vi "Adquisicio_projecte_InsEl (2).vi"() -> ()   [LabVIEW 2014]
uses:
  <vilib>/DAQmx/configure/timing.llb/DAQmx Timing (Sample Clock).vi
  <vilib>/DAQmx/read.llb/DAQmx Read (Analog 1D Wfm NChan NSamp).vi
panel:
  in  "V2":dbl
  in  "V1":dbl
  in  "T2":dbl
  in  "T1":dbl
  in  "Numero de Media":dbl
  in  "Durada adquisició":dbl
  in  "Temps entre adquisicions":dbl
  out "?":bool
  out "?":bool
  out "?":bool
  out "?":bool
  in  "CH 4":bool
  in  "CH 3":bool
  in  "CH 2":bool
  in  "CH 1":bool
  in  "?":bool
  in  "?":bool
  out "Registro Temperatura CH 4":dbl[](graph)
  out "Registro Temperatura CH 3":dbl[](graph)
  out "Registro Temperatura CH 2":dbl[](graph)
  out "Registro Temperatura CH 1":dbl[](graph)
  in  "Tab Control":enum32{"CH 1", "CH 2", "CH 3", "CH 4"}(tab)
  out "T min CH 1":dbl
  out "T max CH 1":dbl
  in  "T max CH 1":dbl
  in  "T min CH 1":dbl
  out "IND CH 1":u32(colorbox)
  out "H CH 1":dbl[](array[numeric])
  out "desviació 1":dbl
  in  "T max CH 2":dbl
  in  "T min CH 2":dbl
  out "IND CH 2":u32(colorbox)
  out "H CH 2":dbl[](array[numeric])
  out "T max CH 2":dbl
  out "T min CH 2":dbl
  in  "T max CH 3":dbl
  in  "T min CH 3":dbl
  out "IND CH 3":u32(colorbox)
  out "H CH 3":dbl[](array[numeric])
  out "T max CH 3":dbl
  out "T min CH 3":dbl
  out "Desviació 3":dbl
  in  "T max CH 4":dbl
  in  "T min CH 4":dbl
  out "IND CH 4":u32(colorbox)
  out "H CH 4":dbl[](array[numeric])
  out "T max CH 4":dbl
  out "T min CH 4":dbl
  out "Desviació 4":dbl
  in  "PARAR PROGRAMA":bool
  out "MEDIA CH 4":dbl
  out "MEDIA CH 3":dbl
  out "MEDIA CH 2":dbl
  out "MEDIA CH 1":dbl
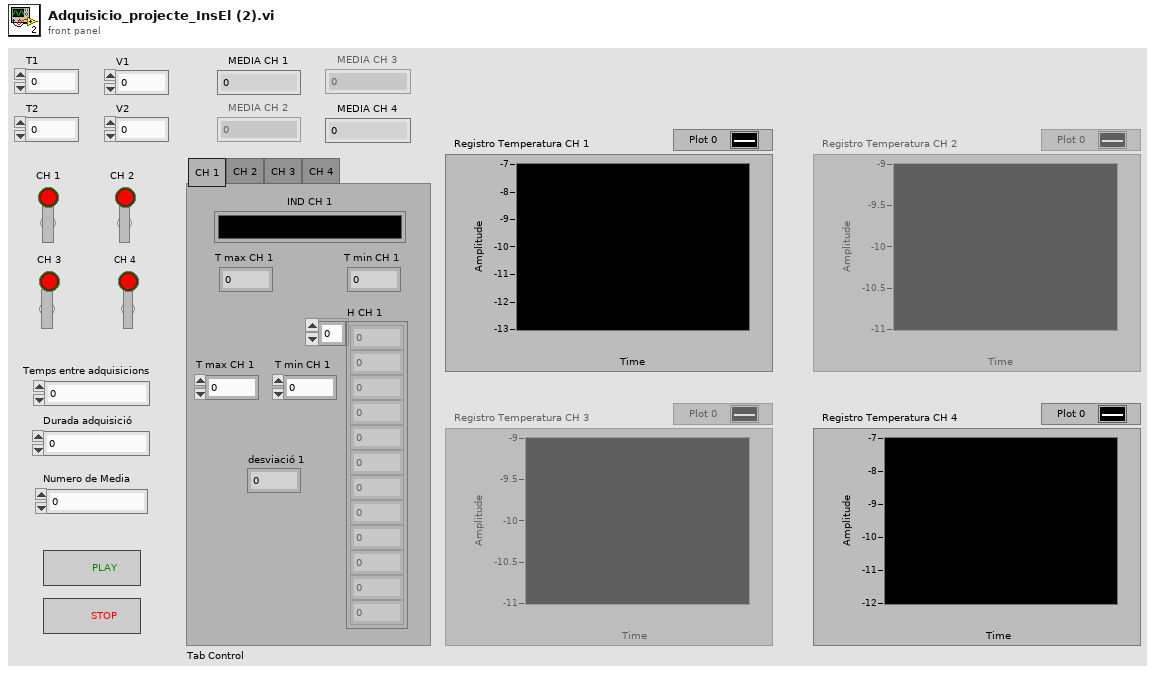
[diagram p1: front panel]
types:
  T1 = enum16{"open", "replace", "create", "open or create", "replace or create", "replace or create with confirmation"}
  T2 = enum8{"Enabled", "Disabled", "Disabled and Grayed Out"}
  T3 = cluster{"CH 1":bool, "CH 2":bool, "CH 3":bool, "CH 4":bool}
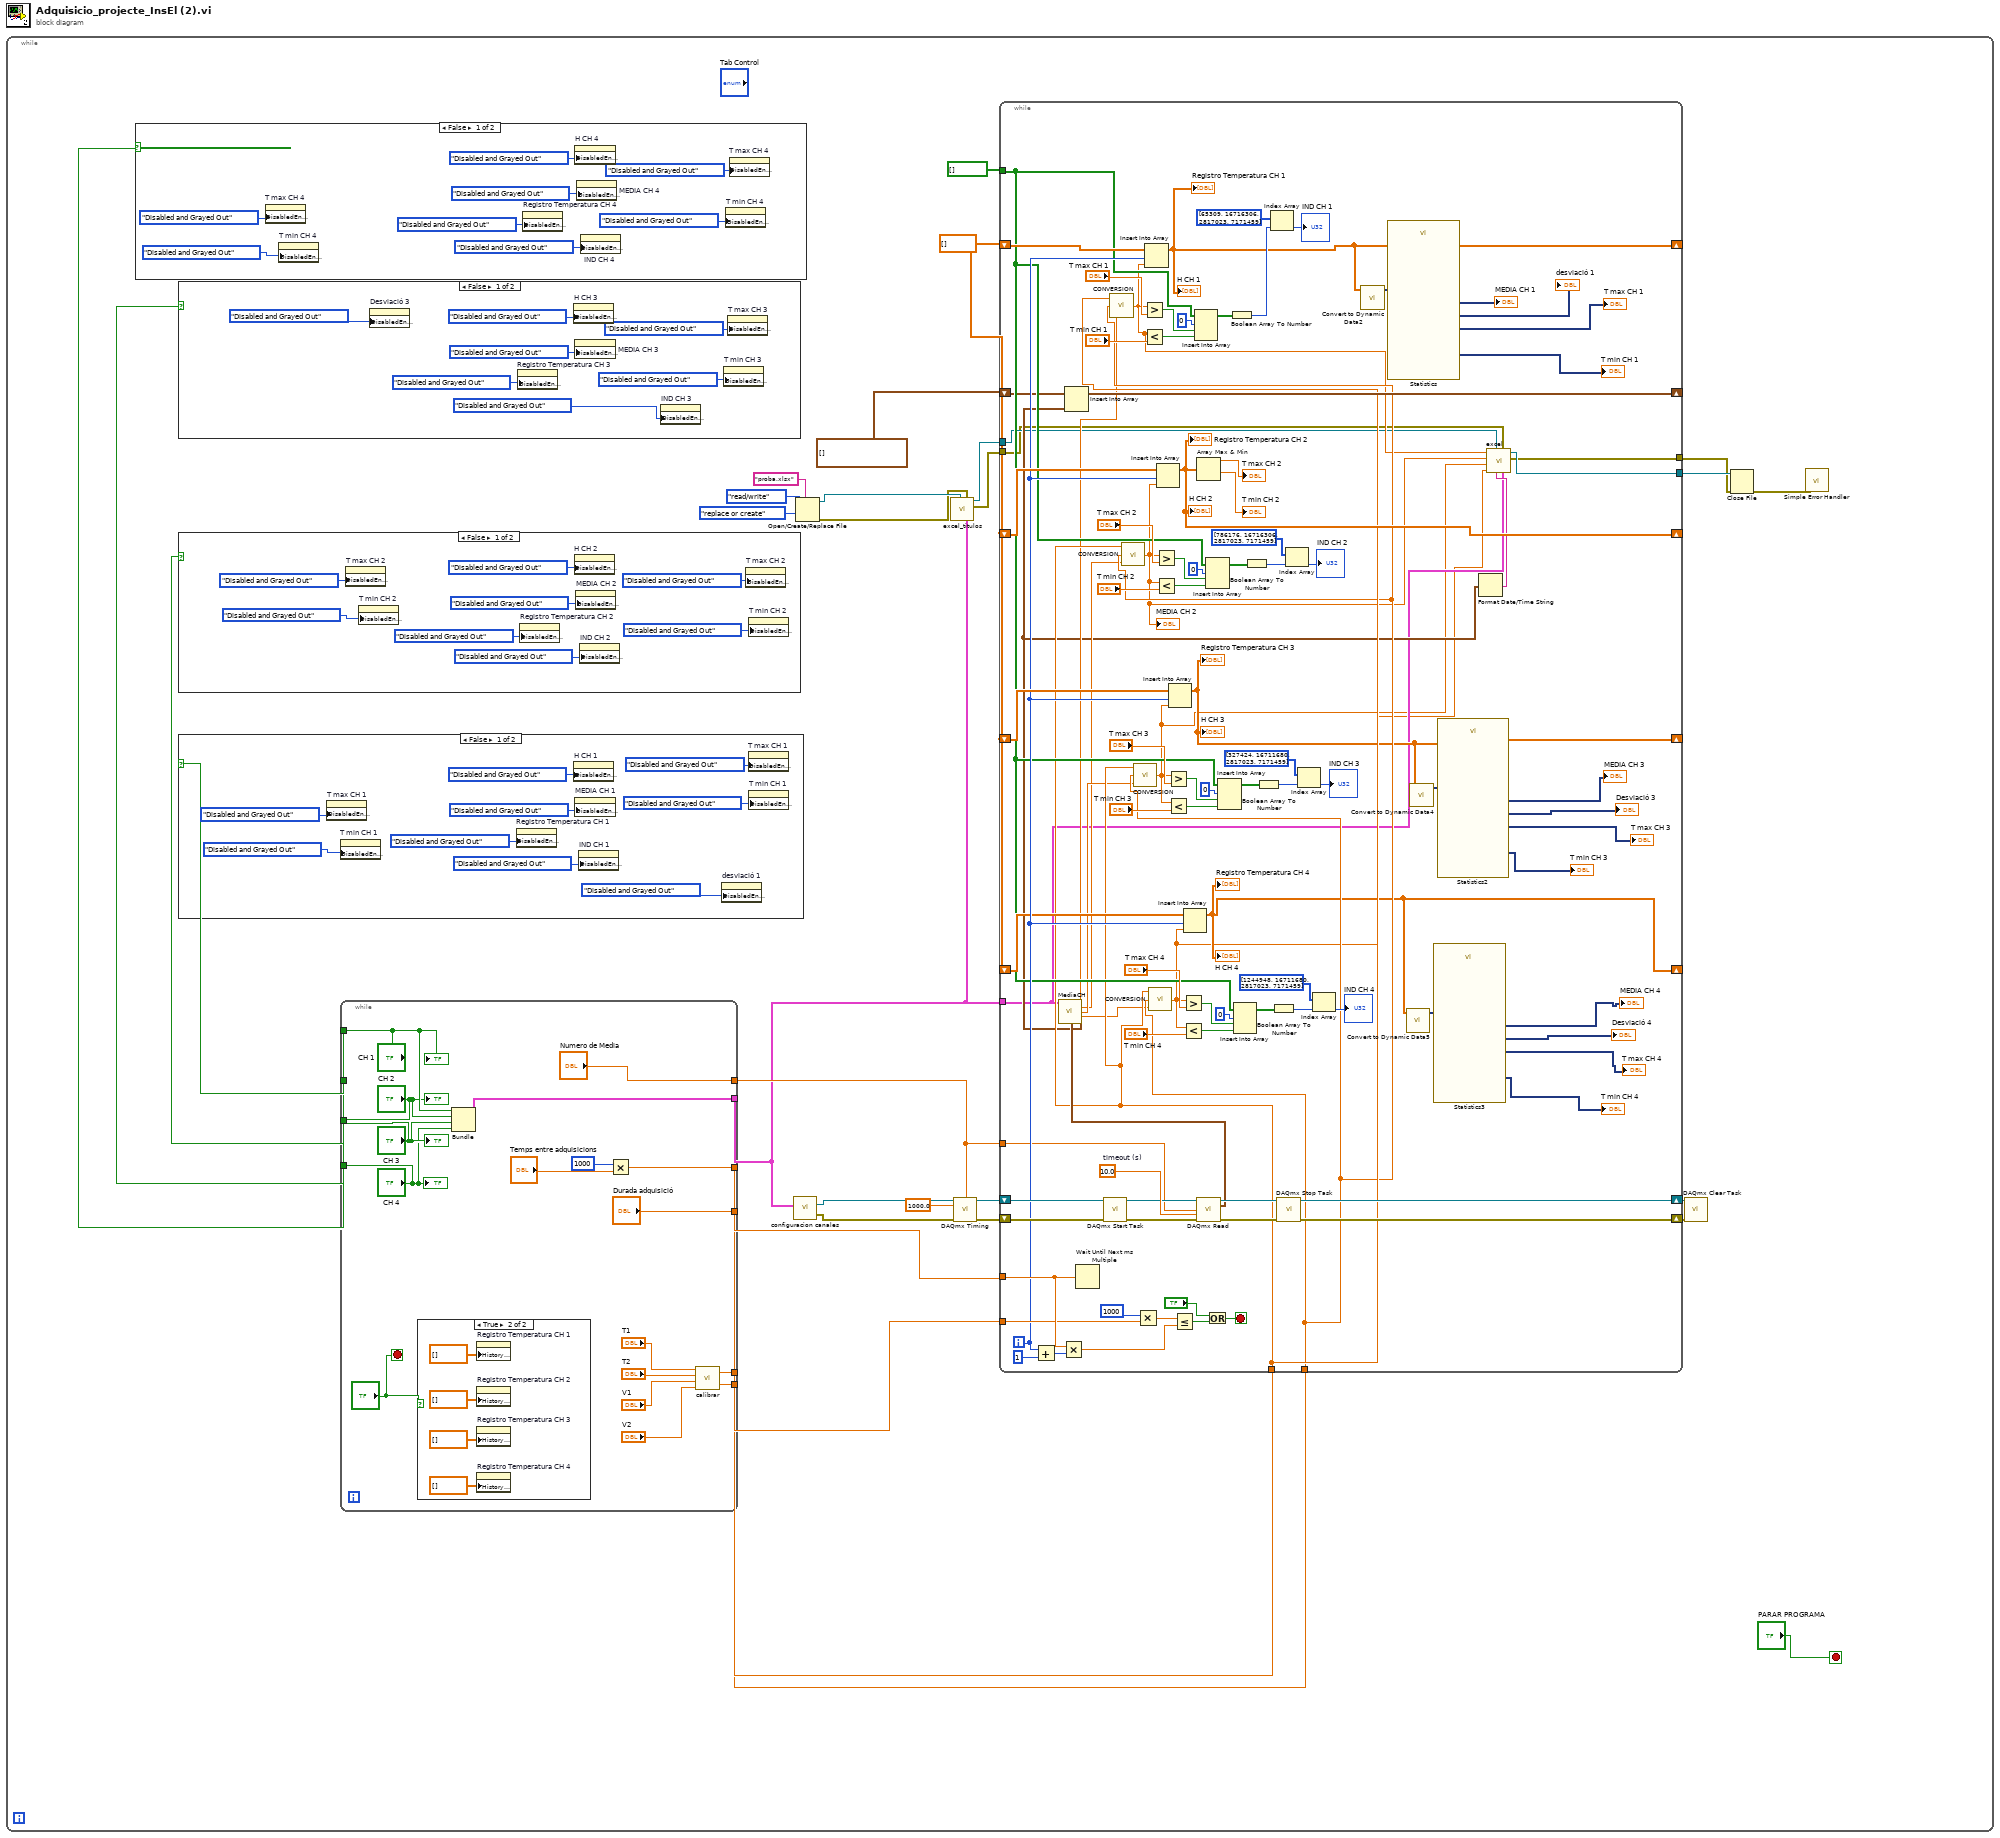
[diagram p0: block diagram]
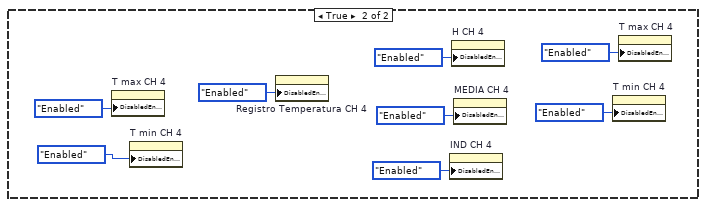
[diagram p2: hidden frame]
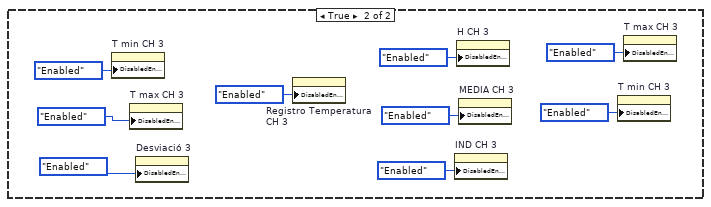
[diagram p3: hidden frame]
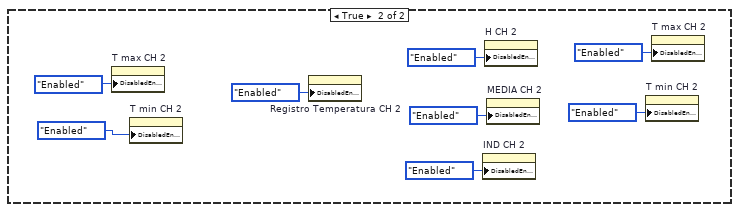
[diagram p4: hidden frame]
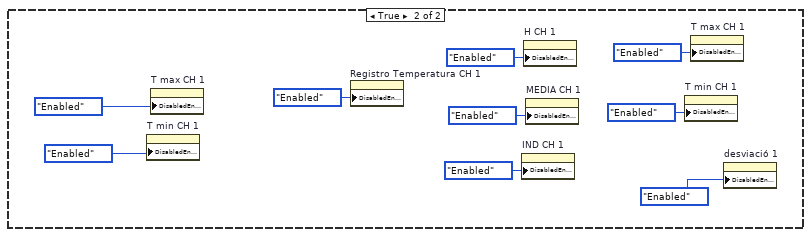
[diagram p5: hidden frame]
diagram:
  n1 = while {
    stop <- "PARAR PROGRAMA" stop-if-true
    w24 = dbl[] [] ("array")
    n2 = while {
      tunnel: [w114] -> w3
      tunnel: ["CH 1"] -> w21
      tunnel: ["CH 2"] -> w18
      tunnel: ["CH 3"] -> w19
      tunnel: ["CH 4"] -> w20
      tunnel: ["Numero de Media"] -> w14
      tunnel: [w105] -> w16
      tunnel: ["Durada adquisició"] -> w15
      tunnel: [w99] -> w13
      tunnel: [w98] -> w12
      stop <- "?" stop-if-true
      n3 = case shown="True" "?" {
        frame False {
        }
        frame True {
          n4 = property on="Registro Temperatura CH 1" class="WFChart (strict)"("History Data"=dbl[] []) -> ()  [unwired: 2 in, 2 out]
          n5 = property on="Registro Temperatura CH 2" class="WFChart (strict)"("History Data"=dbl[] []) -> ()  [unwired: 2 in, 2 out]
          n6 = property on="Registro Temperatura CH 3" class="WFChart (strict)"("History Data"=dbl[] []) -> ()  [unwired: 2 in, 2 out]
          n7 = property on="Registro Temperatura CH 4" class="WFChart (strict)"("History Data"=dbl[] []) -> ()  [unwired: 2 in, 2 out]
        }
      }
      n8 = Bundle("CH 1"="CH 1", "CH 2"="CH 2", "CH 3"="CH 3", "CH 4"="CH 4") -> (w114:T3)  [unwired: 1 in]
      n9 = Multiply(x=1000, y="Temps entre adquisicions") -> (x*y=w105:dbl)
      n10 = call "calibrar.vi"("V 2"="V2", "V1"="V1", "Temp2"="T2", "Temp"="T1") -> ("B"=w98:dbl, "A"=w99:dbl)
      "?" <- "CH 1"
      "?" <- "CH 2"
      "?" <- "CH 3"
      "?" <- "CH 4"
    }
    n11 = case shown="False" w20 {
      frame False {
        n12 = property on="T max CH 4" class="DigNum (strict)"("DisabledEnum"=T2."Disabled and Grayed Out" ("Disabled")) -> ()  [unwired: 2 in, 2 out]
        n13 = property on="T min CH 4" class="DigNum (strict)"("DisabledEnum"=T2."Disabled and Grayed Out" ("Disabled")) -> ()  [unwired: 2 in, 2 out]
        n14 = property on="Registro Temperatura CH 4" class="WFChart (strict)"("DisabledEnum"=T2."Disabled and Grayed Out" ("Disabled")) -> ()  [unwired: 2 in, 2 out]
        n15 = property on="H CH 4" class="Arr (strict)"("DisabledEnum"=T2."Disabled and Grayed Out" ("Disabled")) -> ()  [unwired: 2 in, 2 out]
        n16 = property on="MEDIA CH 4" class="DigNum (strict)"("DisabledEnum"=T2."Disabled and Grayed Out" ("Disabled")) -> ()  [unwired: 2 in, 2 out]
        n17 = property on="IND CH 4" class="ColBox"("DisabledEnum"=T2."Disabled and Grayed Out" ("Disabled")) -> ()  [unwired: 2 in, 2 out]
        n18 = property on="T min CH 4" class="DigNum (strict)"("DisabledEnum"=T2."Disabled and Grayed Out" ("Disabled")) -> ()  [unwired: 2 in, 2 out]
        n19 = property on="T max CH 4" class="DigNum (strict)"("DisabledEnum"=T2."Disabled and Grayed Out" ("Disabled")) -> ()  [unwired: 2 in, 2 out]
      }
      frame True {
        n20 = property on="T max CH 4" class="DigNum (strict)"("DisabledEnum"=T2."Enabled" ("Disabled")) -> ()  [unwired: 2 in, 2 out]
        n21 = property on="T min CH 4" class="DigNum (strict)"("DisabledEnum"=T2."Enabled" ("Disabled")) -> ()  [unwired: 2 in, 2 out]
        n22 = property on="Registro Temperatura CH 4" class="WFChart (strict)"("DisabledEnum"=T2."Enabled" ("Disabled")) -> ()  [unwired: 2 in, 2 out]
        n23 = property on="IND CH 4" class="ColBox"("DisabledEnum"=T2."Enabled" ("Disabled")) -> ()  [unwired: 2 in, 2 out]
        n24 = property on="H CH 4" class="Arr (strict)"("DisabledEnum"=T2."Enabled" ("Disabled")) -> ()  [unwired: 2 in, 2 out]
        n25 = property on="MEDIA CH 4" class="DigNum (strict)"("DisabledEnum"=T2."Enabled" ("Disabled")) -> ()  [unwired: 2 in, 2 out]
        n26 = property on="T min CH 4" class="DigNum (strict)"("DisabledEnum"=T2."Enabled" ("Disabled")) -> ()  [unwired: 2 in, 2 out]
        n27 = property on="T max CH 4" class="DigNum (strict)"("DisabledEnum"=T2."Enabled" ("Disabled")) -> ()  [unwired: 2 in, 2 out]
      }
    }
    n28 = case shown="False" w19 {
      frame False {
        n29 = property on="Desviació 3" class="DigNum (strict)"("DisabledEnum"=T2."Disabled and Grayed Out" ("Disabled")) -> ()  [unwired: 2 in, 2 out]
        n30 = property on="Registro Temperatura CH 3" class="WFChart (strict)"("DisabledEnum"=T2."Disabled and Grayed Out" ("Disabled")) -> ()  [unwired: 2 in, 2 out]
        n31 = property on="H CH 3" class="Arr (strict)"("DisabledEnum"=T2."Disabled and Grayed Out" ("Disabled")) -> ()  [unwired: 2 in, 2 out]
        n32 = property on="MEDIA CH 3" class="DigNum (strict)"("DisabledEnum"=T2."Disabled and Grayed Out" ("Disabled")) -> ()  [unwired: 2 in, 2 out]
        n33 = property on="IND CH 3" class="ColBox"("DisabledEnum"=T2."Disabled and Grayed Out" ("Disabled")) -> ()  [unwired: 2 in, 2 out]
        n34 = property on="T min CH 3" class="DigNum (strict)"("DisabledEnum"=T2."Disabled and Grayed Out" ("Disabled")) -> ()  [unwired: 2 in, 2 out]
        n35 = property on="T max CH 3" class="DigNum (strict)"("DisabledEnum"=T2."Disabled and Grayed Out" ("Disabled")) -> ()  [unwired: 2 in, 2 out]
      }
      frame True {
        n36 = property on="T min CH 3" class="DigNum (strict)"("DisabledEnum"=T2."Enabled" ("Disabled")) -> ()  [unwired: 2 in, 2 out]
        n37 = property on="T max CH 3" class="DigNum (strict)"("DisabledEnum"=T2."Enabled" ("Disabled")) -> ()  [unwired: 2 in, 2 out]
        n38 = property on="Desviació 3" class="DigNum (strict)"("DisabledEnum"=T2."Enabled" ("Disabled")) -> ()  [unwired: 2 in, 2 out]
        n39 = property on="Registro Temperatura CH 3" class="WFChart (strict)"("DisabledEnum"=T2."Enabled" ("Disabled")) -> ()  [unwired: 2 in, 2 out]
        n40 = property on="IND CH 3" class="ColBox"("DisabledEnum"=T2."Enabled" ("Disabled")) -> ()  [unwired: 2 in, 2 out]
        n41 = property on="H CH 3" class="Arr (strict)"("DisabledEnum"=T2."Enabled" ("Disabled")) -> ()  [unwired: 2 in, 2 out]
        n42 = property on="MEDIA CH 3" class="DigNum (strict)"("DisabledEnum"=T2."Enabled" ("Disabled")) -> ()  [unwired: 2 in, 2 out]
        n43 = property on="T min CH 3" class="DigNum (strict)"("DisabledEnum"=T2."Enabled" ("Disabled")) -> ()  [unwired: 2 in, 2 out]
        n44 = property on="T max CH 3" class="DigNum (strict)"("DisabledEnum"=T2."Enabled" ("Disabled")) -> ()  [unwired: 2 in, 2 out]
      }
    }
    n45 = case shown="False" w18 {
      frame False {
        n46 = property on="T max CH 2" class="DigNum (strict)"("DisabledEnum"=T2."Disabled and Grayed Out" ("Disabled")) -> ()  [unwired: 2 in, 2 out]
        n47 = property on="T min CH 2" class="DigNum (strict)"("DisabledEnum"=T2."Disabled and Grayed Out" ("Disabled")) -> ()  [unwired: 2 in, 2 out]
        n48 = property on="Registro Temperatura CH 2" class="WFChart (strict)"("DisabledEnum"=T2."Disabled and Grayed Out" ("Disabled")) -> ()  [unwired: 2 in, 2 out]
        n49 = property on="H CH 2" class="Arr (strict)"("DisabledEnum"=T2."Disabled and Grayed Out" ("Disabled")) -> ()  [unwired: 2 in, 2 out]
        n50 = property on="MEDIA CH 2" class="DigNum (strict)"("DisabledEnum"=T2."Disabled and Grayed Out" ("Disabled")) -> ()  [unwired: 2 in, 2 out]
        n51 = property on="IND CH 2" class="ColBox"("DisabledEnum"=T2."Disabled and Grayed Out" ("Disabled")) -> ()  [unwired: 2 in, 2 out]
        n52 = property on="T max CH 2" class="DigNum (strict)"("DisabledEnum"=T2."Disabled and Grayed Out" ("Disabled")) -> ()  [unwired: 2 in, 2 out]
        n53 = property on="T min CH 2" class="DigNum (strict)"("DisabledEnum"=T2."Disabled and Grayed Out" ("Disabled")) -> ()  [unwired: 2 in, 2 out]
      }
      frame True {
        n54 = property on="T max CH 2" class="DigNum (strict)"("DisabledEnum"=T2."Enabled" ("Disabled")) -> ()  [unwired: 2 in, 2 out]
        n55 = property on="T min CH 2" class="DigNum (strict)"("DisabledEnum"=T2."Enabled" ("Disabled")) -> ()  [unwired: 2 in, 2 out]
        n56 = property on="Registro Temperatura CH 2" class="WFChart (strict)"("DisabledEnum"=T2."Enabled" ("Disabled")) -> ()  [unwired: 2 in, 2 out]
        n57 = property on="IND CH 2" class="ColBox"("DisabledEnum"=T2."Enabled" ("Disabled")) -> ()  [unwired: 2 in, 2 out]
        n58 = property on="H CH 2" class="Arr (strict)"("DisabledEnum"=T2."Enabled" ("Disabled")) -> ()  [unwired: 2 in, 2 out]
        n59 = property on="MEDIA CH 2" class="DigNum (strict)"("DisabledEnum"=T2."Enabled" ("Disabled")) -> ()  [unwired: 2 in, 2 out]
        n60 = property on="T min CH 2" class="DigNum (strict)"("DisabledEnum"=T2."Enabled" ("Disabled")) -> ()  [unwired: 2 in, 2 out]
        n61 = property on="T max CH 2" class="DigNum (strict)"("DisabledEnum"=T2."Enabled" ("Disabled")) -> ()  [unwired: 2 in, 2 out]
      }
    }
    n62 = case shown="False" w21 {
      frame False {
        n63 = property on="T max CH 1" class="DigNum (strict)"("DisabledEnum"=T2."Disabled and Grayed Out" ("Disabled")) -> ()  [unwired: 2 in, 2 out]
        n64 = property on="T min CH 1" class="DigNum (strict)"("DisabledEnum"=T2."Disabled and Grayed Out" ("Disabled")) -> ()  [unwired: 2 in, 2 out]
        n65 = property on="Registro Temperatura CH 1" class="WFChart (strict)"("DisabledEnum"=T2."Disabled and Grayed Out" ("Disabled")) -> ()  [unwired: 2 in, 2 out]
        n66 = property on="H CH 1" class="Arr (strict)"("DisabledEnum"=T2."Disabled and Grayed Out" ("Disabled")) -> ()  [unwired: 2 in, 2 out]
        n67 = property on="MEDIA CH 1" class="DigNum (strict)"("DisabledEnum"=T2."Disabled and Grayed Out" ("Disabled")) -> ()  [unwired: 2 in, 2 out]
        n68 = property on="IND CH 1" class="ColBox"("DisabledEnum"=T2."Disabled and Grayed Out" ("Disabled")) -> ()  [unwired: 2 in, 2 out]
        n69 = property on="desviació 1" class="DigNum (strict)"("DisabledEnum"=T2."Disabled and Grayed Out" ("Disabled")) -> ()  [unwired: 2 in, 2 out]
        n70 = property on="T max CH 1" class="DigNum (strict)"("DisabledEnum"=T2."Disabled and Grayed Out" ("Disabled")) -> ()  [unwired: 2 in, 2 out]
        n71 = property on="T min CH 1" class="DigNum (strict)"("DisabledEnum"=T2."Disabled and Grayed Out" ("Disabled")) -> ()  [unwired: 2 in, 2 out]
      }
      frame True {
        n72 = property on="T min CH 1" class="DigNum (strict)"("DisabledEnum"=T2."Enabled" ("Disabled")) -> ()  [unwired: 2 in, 2 out]
        n73 = property on="T max CH 1" class="DigNum (strict)"("DisabledEnum"=T2."Enabled" ("Disabled")) -> ()  [unwired: 2 in, 2 out]
        n74 = property on="Registro Temperatura CH 1" class="WFChart (strict)"("DisabledEnum"=T2."Enabled" ("Disabled")) -> ()  [unwired: 2 in, 2 out]
        n75 = property on="IND CH 1" class="ColBox"("DisabledEnum"=T2."Enabled" ("Disabled")) -> ()  [unwired: 2 in, 2 out]
        n76 = property on="H CH 1" class="Arr (strict)"("DisabledEnum"=T2."Enabled" ("Disabled")) -> ()  [unwired: 2 in, 2 out]
        n77 = property on="MEDIA CH 1" class="DigNum (strict)"("DisabledEnum"=T2."Enabled" ("Disabled")) -> ()  [unwired: 2 in, 2 out]
        n78 = property on="T min CH 1" class="DigNum (strict)"("DisabledEnum"=T2."Enabled" ("Disabled")) -> ()  [unwired: 2 in, 2 out]
        n79 = property on="T max CH 1" class="DigNum (strict)"("DisabledEnum"=T2."Enabled" ("Disabled")) -> ()  [unwired: 2 in, 2 out]
        n80 = property on="desviació 1" class="DigNum (strict)"("DisabledEnum"=T2."Enabled" ("Disabled")) -> ()  [unwired: 2 in, 2 out]
      }
    }
    n81 = call "configuracion canales.vi"("input cluster"=w3) -> ("error out"=w26:errorcluster, "task out"=w27:refnum<k21>)  [unwired: 3 in]
    n82 = Open/Create/Replace File(prompt="proba.xlsx", operation (0:open)=T1."replace or create", access (0:read/write)=enum16{"read/write", "read-only", "write-only"}."read/write") -> (refnum out=w2:refnum<file>, error out=w1:errorcluster)  [unwired: 3 in, 1 out]
    n83 = call "excel_titulos.vi"("input cluster"=w3, "error out"=w1, "refnum out"=w2) -> ("error in"=w4:errorcluster, "refnum"=w5:refnum<file>)  [unwired: 7 in]
    n84 = call-poly <vilib>:"DAQmx Timing.vi"("task/channels in"=w27, "samples per channel"=w14, "rate"=1000.0, "error in"=w26) -> ("task out"=w29:refnum<k21>, "error out"=w28:errorcluster)  [unwired: 10 in]
    n85 = while {
      shift-right: [w218] -> w31
      shift-left: w29 -> [w214]
      shift-right: [w217] -> w30
      shift-left: w28 -> [w204]
      tunnel: w16 -> [w208]
      tunnel: w3 -> [w127]
      tunnel: w14 -> [w160]
      tunnel: w15 -> [w205]
      shift-right: [w145] -> _
      shift-left: w24 -> [w202]
      shift-right: [w157] -> _
      shift-left: w24 -> [w201]
      shift-right: [w141] -> _
      shift-left: w24 -> [w200]
      shift-right: [w130] -> _
      shift-left: w24 -> [w198]
      tunnel: bool[] [] ("array") -> [w165]
      shift-right: [w154] -> _
      shift-left: timestamp[] [] ("array") -> [w155]
      tunnel: w13 -> [w153]
      tunnel: w12 -> [w152]
      tunnel: [w122] -> w7
      tunnel: [w121] -> w6
      tunnel: w5 -> [w120]
      tunnel: w4 -> [w119]
      i -> [w199]
      stop <- w206 stop-if-true
      w221 = 10.0  # timeout (s)
      n86 = Add(x=w199, y=1 ("x")) -> (x+y=w207:i32)
      n87 = Multiply(x=w208, y=w207) -> (x*y=w209:dbl)
      n88 = Wait Until Next ms Multiple(millisecond multiple=w208) -> ()  [unwired: 1 out]
      n89 = call <vilib>:"DAQmx Start Task.vi"("task/channels in"=w214, "error in"=w204) -> ("task out"=w219:refnum<k21>, "error out"=w220:errorcluster)  [unwired: 12 in]
      n90 = Multiply(x=1000, y=w205) -> (x*y=w211:dbl)
      n91 = Less Or Equal?(x=w211, y=w209) -> (x <= y?=w210:bool)
      n92 = call-poly <vilib>:"DAQmx Read.vi"("task/channels in"=w219, "number of samples per channel"=w160, "timeout"=w221, "error in"=w220) -> ("task out"=w216:refnum<k21>, "data"=w156:waveform(dbl)[], "error out"=w215:errorcluster)  [unwired: 9 in]
      n93 = call "MediaCH.vi"("input cluster"=w127, "Data"=w156) -> ("Mitja CH1"=w148:dbl, "Mitja CH2"=w149:dbl, "Mitja CH3"=w150:dbl, "Mitja CH4"=w151:dbl, "Time Stamp"=w129:timestamp)  [unwired: 9 in]
      n94 = Insert Into Array(array=w155, new element=w129) -> (w154:timestamp[])  [unwired: 1 in]
      n95 = call "CONVERSION.vi"("V1"=w148, "B"=w152, "A"=w153) -> ("Temp"=w126:dbl)
      n96 = call "CONVERSION.vi"("V1"=w149, "B"=w152, "A"=w153) -> ("Temp"=w125:dbl)
      "MEDIA CH 2" <- w125
      n97 = call "CONVERSION.vi"("V1"=w150, "B"=w152, "A"=w153) -> ("Temp"=w124:dbl)
      n98 = Greater?(x=w126, y="T max CH 1") -> (0:w195:bool)
      n99 = Less?(x=w126, y="T min CH 1") -> (x < y?=w194:bool)
      n100 = Insert Into Array(array=w202, index=w199, new element=w126) -> (w145:dbl[])
      "H CH 1" <- w145
      "Registro Temperatura CH 1" <- w145
      n101 = call "CONVERSION.vi"("V1"=w151, "B"=w152, "A"=w153) -> ("Temp"=w123:dbl)
      n102 = Greater?(x=w125, y="T max CH 2") -> (0:w187:bool)
      n103 = Less?(x=w125, y="T min CH 2") -> (x < y?=w186:bool)
      n104 = Insert Into Array(array=w201, index=w199, new element=w125) -> (w157:dbl[])
      "H CH 2" <- w157
      "Registro Temperatura CH 2" <- w157
      n105 = Greater?(x=w124, y="T max CH 3") -> (0:w180:bool)
      n106 = Less?(x=w124, y="T min CH 3") -> (x < y?=w179:bool)
      n107 = Insert Into Array(array=w200, index=w199, new element=w124) -> (w141:dbl[])
      "H CH 3" <- w141
      "Registro Temperatura CH 3" <- w141
      n108 = Greater?(x=w123, y="T max CH 4") -> (0:w172:bool)
      n109 = Less?(x=w123, y="T min CH 4") -> (x < y?=w171:bool)
      n110 = Insert Into Array(array=w198, index=w199, new element=w123) -> (w130:dbl[])
      "H CH 4" <- w130
      "Registro Temperatura CH 4" <- w130
      n111 = Insert Into Array(array=w165, index=0, new element #1=w195, new element #2=w194) -> (w192:bool[])
      n112 = Array Max & Min(array=w157) -> (max value=→"T max CH 2":dbl, min value=→"T min CH 2":dbl)  [unwired: 2 out]
      n113 = Insert Into Array(array=w165, index=0, new element #1=w187, new element #2=w186) -> (w184:bool[])
      n114 = Or(x="?", y=w210) -> (x .or. y?=w206:bool)
      n115 = Insert Into Array(array=w165, index=0, new element #1=w180, new element #2=w179) -> (w177:bool[])
      n116 = Boolean Array To Number(Boolean array=w192) -> (number=w190:u32)
      n117 = Insert Into Array(array=w165, index=0, new element #1=w172, new element #2=w171) -> (w169:bool[])
      n118 = Boolean Array To Number(Boolean array=w184) -> (number=w182:u32)
      n119 = Boolean Array To Number(Boolean array=w177) -> (number=w175:u32)
      n120 = Index Array(array=u32[] [65309, 16716306, 2817023, 7171459], index=w190) -> (element=→"IND CH 1":u32)
      n121 = Boolean Array To Number(Boolean array=w169) -> (number=w166:u32)
      n122 = call <vilib>:"DAQmx Stop Task.vi"("task/channels in"=w216, "error in"=w215) -> ("task out"=w218:refnum<k21>, "error out"=w217:errorcluster)  [unwired: 12 in]
      n123 = Index Array(array=u32[] [786176, 16716306, 2817023, 7171459], index=w182) -> (element=→"IND CH 2":u32)
      n124 = Index Array(array=u32[] [327424, 16711680, 2817023, 7171459], index=w175) -> (element=→"IND CH 3":u32)
      n125 = Index Array(array=u32[] [1244948, 16711680, 2817023, 7171459], index=w166) -> (element=→"IND CH 4":u32)
      n126 = call "Convert to Dynamic Data2"("Array"=w145) -> ("Dynamic Data Type"=w144:dynamicdata)  [unwired: 3 in]
      n127 = call "Statistics"("Signals"=w144) -> ("Standard Dev"=→"desviació 1":dynamicdata, "Arithmetic Mean"=→"MEDIA CH 1":dynamicdata, "Minimum"=→"T min CH 1":dynamicdata, "Maximum"=→"T max CH 1":dynamicdata)  [unwired: 20 in, 3 out]
      n128 = call "Convert to Dynamic Data5"("Array"=w130) -> ("Dynamic Data Type"=w135:dynamicdata)  [unwired: 3 in]
      n129 = call "Convert to Dynamic Data4"("Array"=w141) -> ("Dynamic Data Type"=w140:dynamicdata)  [unwired: 3 in]
      n130 = call "Statistics3"("Signals"=w135) -> ("Standard Dev"=→"Desviació 4":dynamicdata, "Arithmetic Mean"=→"MEDIA CH 4":dynamicdata, "Minimum"=→"T min CH 4":dynamicdata, "Maximum"=→"T max CH 4":dynamicdata)  [unwired: 20 in, 3 out]
      n131 = call "Statistics2"("Signals"=w140) -> ("Standard Dev"=→"Desviació 3":dynamicdata, "Arithmetic Mean"=→"MEDIA CH 3":dynamicdata, "Minimum"=→"T min CH 3":dynamicdata, "Maximum"=→"T max CH 3":dynamicdata)  [unwired: 20 in, 3 out]
      n132 = Format Date/Time String(seconds (now)=w129) -> (date/time string=w128:string)  [unwired: 2 in]
      n133 = call "excel.vi"("input cluster"=w127, "error out"=w119, "fecha y hora"=w128, "refnum out"=w120, "CH 4"=w123, "CH 3"=w124, "CH 2"=w125, "CH 1"=w126) -> ("error in"=w121:errorcluster, "refnum"=w122:refnum<file>)  [unwired: 2 in]
    }
    n134 = call <vilib>:"DAQmx Clear Task.vi"("task in"=w31, "error in"=w30) -> ()  [unwired: 13 in, 1 out]
    n135 = Close File(refnum=w7, error in=w6) -> (error out=w11:errorcluster)  [unwired: 1 out]
    n136 = call <vilib>:"Simple Error Handler.vi"("error in (no error)"=w11) -> ()  [unwired: 4 in, 5 out]
  }
